vi "Do.vi"(8 "error in (no error)":errorcluster, 10 "Actor in":refnum<class "Actor.lvclass">, 11 "Handle Mouse Down Msg":refnum<class "Handle Mouse Down Msg.lvclass">) -> (0 "error out":errorcluster, 2 "Actor out":refnum<class "Actor.lvclass">)   [LabVIEW 2017, in "Handle Mouse Down Msg.lvclass"]
doc: "This VI delivers the message to the actor by calling the appropriate method(s) on the actor."
uses:
  <vilib>/gpm_packages/@cs/Test-executive-builder/Source/Test Executive Builder View/Test Executive Builder View Messages/Handle Mouse Down Msg/Handle Mouse Down Msg.lvclass
  <vilib>/ActorFramework/Actor/Actor.lvclass
  <vilib>/gpm_packages/@cs/Test-executive-builder/Source/Test Executive Builder View/Test Executive Builder View/Test Executive Builder View.lvclass
  C:/Program Files/National Instruments/LabVIEW 2017/vi.lib/ActorFramework/Actor/Actor.lvclass
  <vilib>/gpm_packages/@cs/Test-executive-builder/Source/Test Executive Builder View/Test Executive Builder View Messages/Handle Mouse Down Msg/Handle Mouse Down Msg.lvclass/Handle Mouse Down Msg.ctl
  <vilib>/gpm_packages/@cs/Test-executive-builder/Source/Application Dependencies/Mouse Down Filtered Event Data.ctl
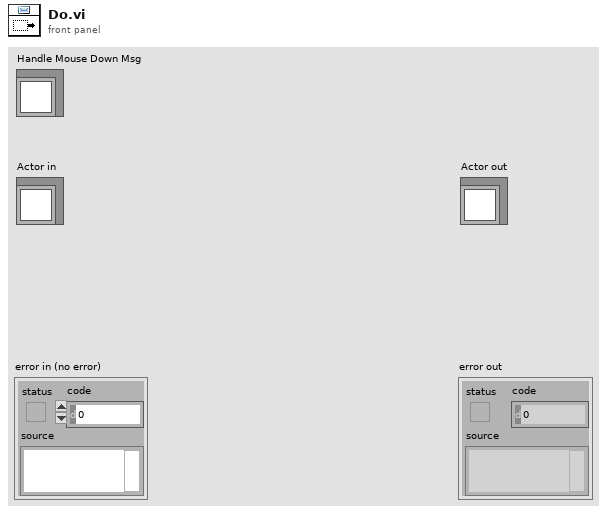
[diagram p1: front panel]
types:
  T1 = typedef "LVPoint32TypeDef.ctl" = cluster{"Horizontal":i32, "Vertical":i32}
  T2 = cluster{"Shift":bool, "Ctrl":bool, "Alt":bool, "Cmd":bool, "Opt":bool}
  T3 = typedef "Mouse Down Filtered Event Data.ctl" = cluster{"Button":u16, "Mods":cluster{"Num Pad":bool, "Menu Key":bool}, "PlatMods":cluster{"Shift":bool, "Ctrl":bool, "Alt":bool, "Cmd":bool, "Opt":bool}, "Data Filtered?":bool, "Discard?":bool}
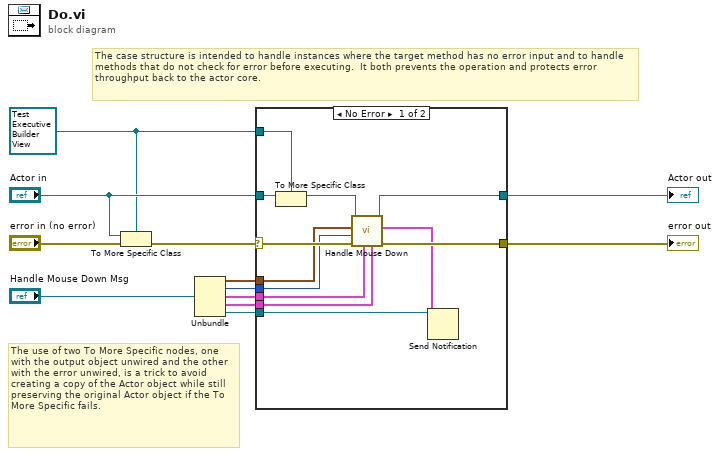
[diagram p0: block diagram]
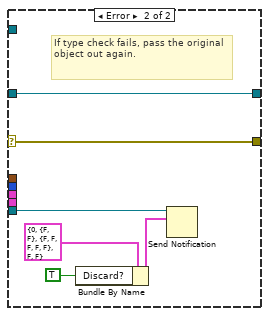
[diagram p2: hidden frame]
diagram:
  w6 = refnum<class "Test Executive Builder View.lvclass"> refnum ("Actor in")
  # "The use of two To More Specific nodes, one with the output object unwired and the other with the error unwired, is a trick to avoid creating a copy of the Actor object while still preserving the original Actor object if the To More Specific fails."
  # "The case structure is intended to handle instances where the target method has no error input and to handle methods that do not check for error before executing.  It both prevents the operation and protects error throughput back to the actor core."
  n1 = To More Specific Class(target class=w6, reference="Actor in", error in="error in (no error)") -> (error out=w10:errorcluster)  [unwired: 1 out]
  n2 = Unbundle("Handle Mouse Down Msg") -> (w5:T1, w4:u16, w3:cluster{"Double Click":bool, "Menu Key":bool}, w2:T2, w1:refnum<notifier>)
  n3 = case shown="No Error" w10 {
    selector: w10 -> [w22 w30]
    tunnel: [w24 w30] -> w9
    tunnel: [w23 w29] -> w8
    tunnel: "Actor in" -> [w21 w29]
    tunnel: w6 -> [w20 _]
    tunnel: w5 -> [w18 _]
    tunnel: w4 -> [w17 _]
    tunnel: w3 -> [w16 _]
    tunnel: w2 -> [w15 _]
    tunnel: w1 -> [w14 w28]
    frame No Error {
      n4 = To More Specific Class(target class=w20, reference=w21) -> (specific class reference=w19:refnum<class "Test Executive Builder View.lvclass">)  [unwired: 1 in, 1 out]
      n5 = call-dynamic "Handle Mouse Down.vi"("PlatMods"=w15, "Mods"=w16, "error in (no error)"=w22, "Button"=w17, "Coords"=w18, "Test Executive Builder View in"=w19) -> ("error out"=w24:errorcluster, "Mouse Down Filtered Event Data"=w13:T3, "Test Executive Builder View out"=w23:refnum<class "Test Executive Builder View.lvclass">)  [unwired: 3 in]
      n6 = Send Notification(notification=w13, notifier=w14) -> ()  [unwired: 1 in, 2 out]
    }
    frame Error {
      # "If type check fails, pass the original object out again."
      n7 = Bundle By Name(cluster=T3 {"Button"=0, "Mods"={"Num Pad"=FALSE, "Menu Key"=FALSE}, "PlatMods"={"Shift"=FALSE, "Ctrl"=FALSE, "Alt"=FALSE, "Cmd"=FALSE, "Opt"=FALSE}, "Data Filtered?"=FALSE, "Discard?"=FALSE} ("notification"), "Discard?"=TRUE) -> (w25:T3)
      n8 = Send Notification(notification=w25, notifier=w28) -> ()  [unwired: 1 in, 2 out]
    }
  }
  "error out" <- w9
  "Actor out" <- w8
